vi "PH_Beckhoff_StepMot.Motor Type Configuration.vi"(1 "Motor Type":T1) -> (0 "Step Motor Configuration":T2)   [LabVIEW 2014, in "PH_Beckhoff_StepMot.lvlib"]
doc: "This VI contains the Motor parameters. The neutral parameter (when the paramter is not set at all) is typically a \"-1\"."
uses:
  PH_Beckhoff_StepMot.lvlib
  instr.lib/Beckhoff/Specials/Step Motor Klemmen/Beckhoff.Step Motor - Motor Configuration.ctl
  instr.lib/Beckhoff/Read and Write Register/Step Motor Klemmen/Beckhoff.Step Motor - Feature Register 1.ctl
  instr.lib/Beckhoff/Read and Write Register/Step Motor Klemmen/Beckhoff.Step Motor - Feature Register 2.ctl
  PH_Basics/PH_Stepmotor_BaseClass/PH_Stepmotor_BaseClass.Motor Type.ctl
  instr.lib/Beckhoff/Beckhoff - Driver np.lvlib
  PH_Basics/PH_Stepmotor_BaseClass/PH_Stepmotor_BaseClass.lvlib
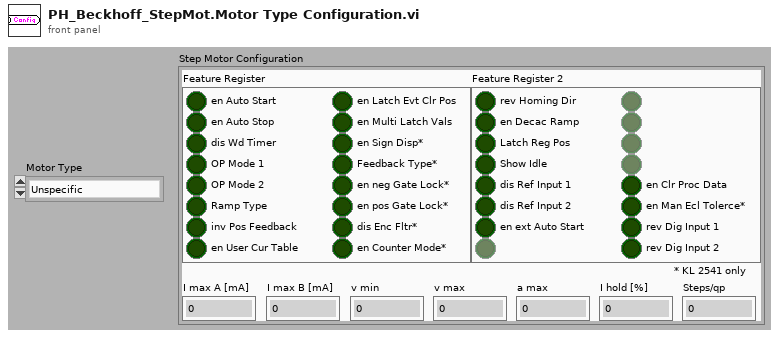
[diagram p1: front panel]
types:
  T1 = typedef "PH_Stepmotor_BaseClass.lvlib/PH_Stepmotor_BaseClass.Motor Type.ctl" = enum16{"Unspecific", "OWIS 49.120.2633", "OWIS 49.060.1033", "OWIS 43.040.2558", "Diamond Motion 2200 series", "OWIS 49.120.266B.MV6", "Calorimeter", "Linear Stage 1", "MICOS VT-80", "MICOS VT-80 S", "Standa Rotstage nt0.95A", "PUF RA 320.200", "PUF RA 800.200", "PUF RA 800.400", "PUF RA 400.50", "1324.nn.800.50", "1324.n9c.800.50", "1324.nn.320.200", "1324.nn.400.200", "1324.nn.800.200", "1324.nn.400.50", "1324.8c9c.800.50", "1324.8c9c.400.200"}
  T2 = typedef "Beckhoff - Driver np.lvlib/Beckhoff.Step Motor - Motor Configuration.ctl" = cluster{"Feature Register":T3, "I max A [mA]":dbl, "I max B [mA]":dbl, "v min":u32, "v max":u32, "a max":u32, "I hold [%]":u32, "Steps/qp":u32, "Feature Register 2":T4}
  T3 = typedef "Beckhoff - Driver np.lvlib/Beckhoff.Step Motor - Feature Register 1.ctl" = cluster{"en Auto Start":bool, "en Auto Stop":bool, "dis Wd Timer":bool, "OP Mode 1":bool, "OP Mode 2":bool, "Ramp Type":bool, "inv Pos Feedback":bool, "en User Cur Table":bool, "en Latch Evt Clr Pos":bool, "en Multi Latch Vals":bool, "en Sign Disp*":bool, "Feedback Type*":bool, "en neg Gate Lock*":bool, "en pos Gate Lock*":bool, "dis Enc Fltr*":bool, "en Counter Mode*":bool}
  T4 = typedef "Beckhoff - Driver np.lvlib/Beckhoff.Step Motor - Feature Register 2.ctl" = cluster{"rev Homing Dir":bool, "en Decac Ramp":bool, "Latch Reg Pos":bool, "Show Idle":bool, "dis Ref Input 1":bool, "dis Ref Input 2":bool, "en ext Auto Start":bool, "N/A":bool, "N/A":bool, "N/A":bool, "N/A":bool, "N/A":bool, "en Clr Proc Data":bool, "en Man Ecl Tolerce*":bool, "rev Dig Input 1":bool, "rev Dig Input 2":bool}
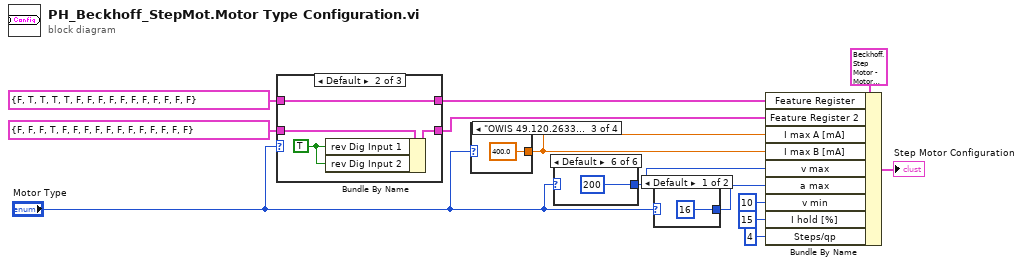
[diagram p0: block diagram]
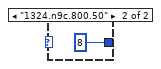
[diagram p2: hidden frame]
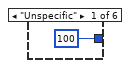
[diagram p3: hidden frame]
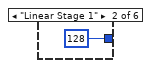
[diagram p4: hidden frame]
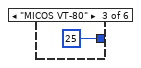
[diagram p5: hidden frame]
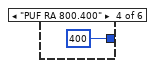
[diagram p6: hidden frame]
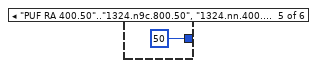
[diagram p7: hidden frame]
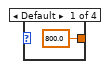
[diagram p8: hidden frame]
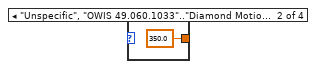
[diagram p9: hidden frame]
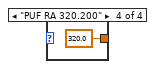
[diagram p10: hidden frame]
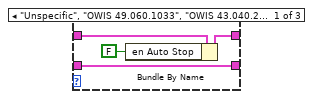
[diagram p11: hidden frame]
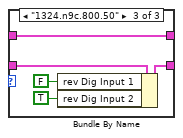
[diagram p12: hidden frame]
diagram:
  n1 = case shown="Default" "Motor Type" {
    tunnel: T4 {"rev Homing Dir"=FALSE, "en Decac Ramp"=FALSE, "Latch Reg Pos"=FALSE, "Show Idle"=TRUE, "dis Ref Input 1"=FALSE, "dis Ref Input 2"=FALSE, "en ext Auto Start"=FALSE, "N/A"=FALSE, "N/A"=FALSE, "N/A"=FALSE, "N/A"=FALSE, "N/A"=FALSE, "en Clr Proc Data"=FALSE, "en Man Ecl Tolerce*"=FALSE, "rev Dig Input 1"=FALSE, "rev Dig Input 2"=FALSE} ("Feature Register 2") -> [w17 w21 w26]
    tunnel: [w17 w20 w25] -> w8
    tunnel: [w15 w18 w22] -> w6
    tunnel: T3 {"en Auto Start"=FALSE, "en Auto Stop"=TRUE, "dis Wd Timer"=TRUE, "OP Mode 1"=TRUE, "OP Mode 2"=TRUE, "Ramp Type"=FALSE, "inv Pos Feedback"=FALSE, "en User Cur Table"=FALSE, "en Latch Evt Clr Pos"=FALSE, "en Multi Latch Vals"=FALSE, "en Sign Disp*"=FALSE, "Feedback Type*"=FALSE, "en neg Gate Lock*"=FALSE, "en pos Gate Lock*"=FALSE, "dis Enc Fltr*"=FALSE, "en Counter Mode*"=FALSE} ("Feature Register") -> [w16 w18 w22]
    frame "Unspecific", "OWIS 49.060.1033", "OWIS 43.040.2558", "Standa Rotstage nt0.95A", "1324.nn.800.50", "1324.nn.320.200".."1324.nn.400.50" {
      n2 = Bundle By Name(cluster=w16, "en Auto Stop"=FALSE) -> (w15:T3)
    }
    frame Default {
      w19 = TRUE ("rev Dig Input 1")
      n3 = Bundle By Name(cluster=w21, "rev Dig Input 1"=w19, "rev Dig Input 2"=w19) -> (w20:T4)
    }
    frame "1324.n9c.800.50" {
      n4 = Bundle By Name(cluster=w26, "rev Dig Input 1"=FALSE, "rev Dig Input 2"=TRUE ("rev Dig Input 1")) -> (w25:T4)
    }
  }
  n5 = case shown="\"OWIS 49.120.2633\", \"OWIS 49.120.266B.MV6\", \"MICOS VT-80\", \"PUF RA 400.50\", \"1324.nn.400.200\", \"1324.nn.400.50\", \"1324.8c9c.400.200\"" "Motor Type" {
    tunnel: [800.0 ("I max A [mA]") 350.0 ("I max A [mA]") 400.0 ("I max A [mA]") 320.0 ("I max A [mA]")] -> w4
    frame Default {
    }
    frame "Unspecific", "OWIS 49.060.1033".."Diamond Motion 2200 series" {
    }
    frame "OWIS 49.120.2633", "OWIS 49.120.266B.MV6", "MICOS VT-80", "PUF RA 400.50", "1324.nn.400.200", "1324.nn.400.50", "1324.8c9c.400.200" {
    }
    frame "PUF RA 320.200" {
    }
  }
  n6 = case shown="Default" "Motor Type" {
    tunnel: [u32 100 ("v max") u32 128 ("v max") u32 25 ("v max") u32 400 ("v max") u32 50 ("v max") u32 200 ("v max")] -> w3
    frame "Unspecific" {
    }
    frame "Linear Stage 1" {
    }
    frame "MICOS VT-80" {
    }
    frame "PUF RA 800.400" {
    }
    frame "PUF RA 400.50".."1324.n9c.800.50", "1324.nn.400.50", "1324.8c9c.800.50" {
    }
    frame Default {
    }
  }
  n7 = case shown="Default" "Motor Type" {
    tunnel: [u32 16 ("a max") u32 8 ("a max")] -> w2
    frame Default {
    }
    frame "1324.n9c.800.50" {
    }
  }
  n8 = Bundle By Name(cluster=T2 {"Feature Register"={"en Auto Start"=FALSE, "en Auto Stop"=FALSE, "dis Wd Timer"=FALSE, "OP Mode 1"=FALSE, "OP Mode 2"=FALSE, "Ramp Type"=FALSE, "inv Pos Feedback"=FALSE, "en User Cur Table"=FALSE, "en Latch Evt Clr Pos"=FALSE, "en Multi Latch Vals"=FALSE, "en Sign Disp*"=FALSE, "Feedback Type*"=FALSE, "en neg Gate Lock*"=FALSE, "en pos Gate Lock*"=FALSE, "dis Enc Fltr*"=FALSE, "en Counter Mode*"=FALSE}, "I max A [mA]"=0.0, "I max B [mA]"=0.0, "v min"=0, "v max"=0, "a max"=0, "I hold [%]"=0, "Steps/qp"=0, "Feature Register 2"={"rev Homing Dir"=FALSE, "en Decac Ramp"=FALSE, "Latch Reg Pos"=FALSE, "Show Idle"=FALSE, "dis Ref Input 1"=FALSE, "dis Ref Input 2"=FALSE, "en ext Auto Start"=FALSE, "N/A"=FALSE, "N/A"=FALSE, "N/A"=FALSE, "N/A"=FALSE, "N/A"=FALSE, "en Clr Proc Data"=FALSE, "en Man Ecl Tolerce*"=FALSE, "rev Dig Input 1"=FALSE, "rev Dig Input 2"=FALSE}} ("Step Motor Configuration"), "Feature Register"=w6, "Feature Register 2"=w8, "I max A [mA]"=w4, "I max B [mA]"=w4, "v max"=w3, "a max"=w2, "v min"=u32 10 ("v min [%]"), "I hold [%]"=u32 15, "Steps/qp"=u32 4) -> (→"Step Motor Configuration":T2)
